vi "Create pre-empt.vi"(8 "error in (no error)":errorcluster, 11 "_Popup in":refnum<class "Popup.lvclass">) -> (0 "error out":errorcluster, 3 "_Popup out":refnum<class "Popup.lvclass">)   [LabVIEW 2021, in "Pop-Up.lvlib" / "Popup.lvclass"]
doc: "get the pre-emptible notifier reference\n\n<b>Code Developed By:</b> +\nDaniel Coons +\nhttps://github.com/danielcoons/tsc-pop-up"
uses:
  Popup.lvclass
  Popup.lvclass/Popup.ctl
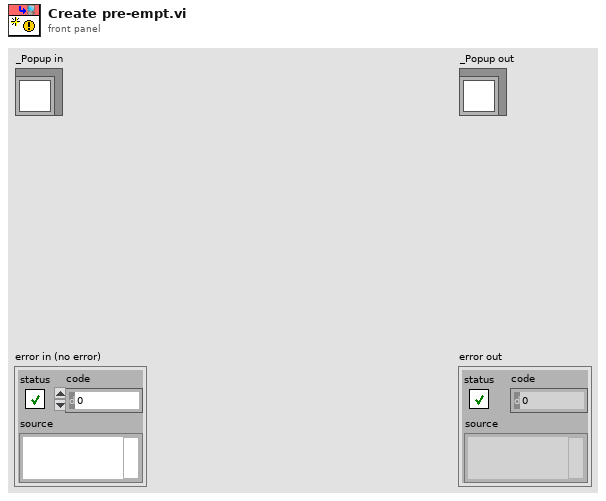
[diagram p1: front panel]
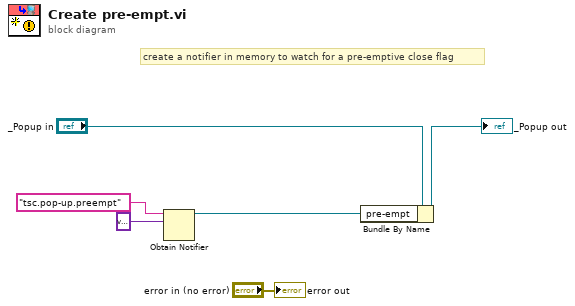
[diagram p0: block diagram]
diagram:
  # "create a notifier in memory to watch for a pre-emptive close flag"
  n1 = Obtain Notifier(name (unnamed)="tsc.pop-up.preempt", notification data type=variant) -> (notifier out=w1:refnum<notifier>)  [unwired: 2 in, 2 out]
  n2 = Bundle By Name(cluster="_Popup in", "pre-empt"=w1) -> (→"_Popup out":refnum<class "Popup.lvclass">)
  "error out" <- "error in (no error)"
